vi "SyncPacket.vi"() -> (2 "sync packet array":u8[](array[numeric]), 3 "sync packet":string)   [LabVIEW 2018]
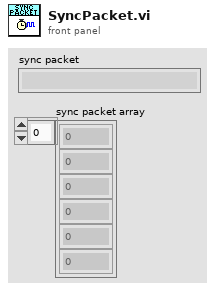
[diagram p1: front panel]
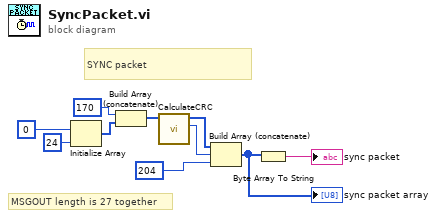
[diagram p0: block diagram]
diagram:
  # "SYNC packet"
  # "MSGOUT length is 27 together"
  n1 = Initialize Array(u8 0, 24 ("dimension size")) -> (w7:u8[])
  n2 = Build Array (concatenate)(u8 170, w7) -> (w8:u8[])
  n3 = call "CalculateCRC.vi"("data in"=w8) -> ("CRC"=w10:u8, "data out"=w9:u8[])  [unwired: 9 in]
  n4 = Build Array (concatenate)(w9, w10, u8 204) -> (w4:u8[])
  "sync packet array" <- w4
  n5 = Byte Array To String(unsigned byte array=w4) -> (string=→"sync packet":string)
